vi "Address API.vi"(8 "error in":errorcluster, 11 "DVR":refnum<data-value>) -> (0 "error out":errorcluster, 3 "DVR Out":refnum<data-value>)   [LabVIEW 2020, in "Speed Mode.lvclass"]
uses:
  Speed Mode.lvclass
  Address/Address.lvclass
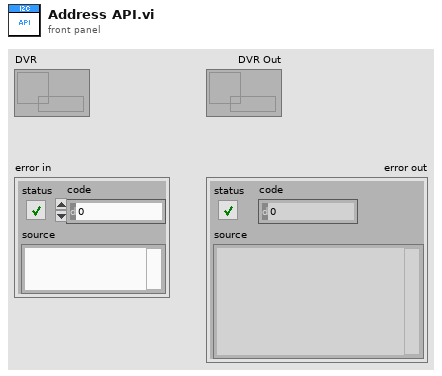
[diagram p1: front panel]
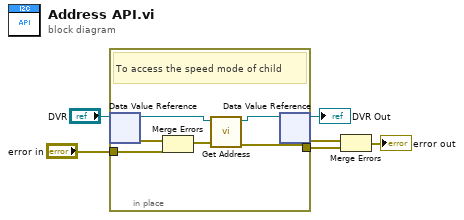
[diagram p0: block diagram]
diagram:
  n1 = in-place {
    in-place-border: "error in" -> [w11]
    in-place-border: [w9] -> w5
    # "To access the speed mode of child"
    n2 = in-place-dvr #1("DVR") -> (w8:refnum<class "Address.lvclass">, w12:errorcluster)
    n3 = Merge Errors(w12, w11) -> (w10:errorcluster)
    n4 = call-dynamic "Get Address.vi"("Error in"=w10, "Address in"=w8) -> ("Error out"=w9:errorcluster, "Address out"=w7:refnum<class "Address.lvclass">)  [unwired: 8 in]
    n5 = in-place-dvr #1(w7) -> (→"DVR Out":refnum<data-value>, w4:errorcluster)
  }
  n6 = Merge Errors(w4, w5) -> (→"error out":errorcluster)
